vi "Set Hardware Info.vi"(10 "Hardware Info":refnum<class "Hardware Info.lvclass">, 11 "Framework in":refnum<class "Framework.lvclass">) -> (3 "Framework out":refnum<class "Framework.lvclass">)   [LabVIEW 2017, in "DSF Core.lvlib" / "Framework.lvclass"]
uses:
  Framework.lvclass
  Hardware/Hardware Info/Hardware Info.lvclass
  Framework.lvclass/Framework.ctl
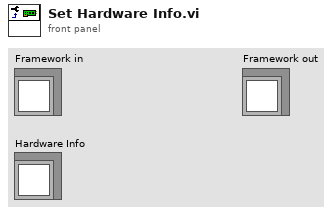
[diagram p1: front panel]
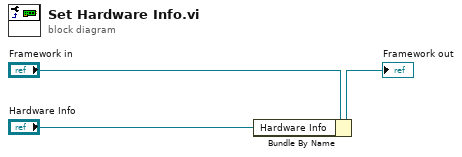
[diagram p0: block diagram]
diagram:
  n1 = Bundle By Name(cluster="Framework in", "Hardware Info"="Hardware Info") -> (→"Framework out":refnum<class "Framework.lvclass">)
